vi "RT_Proof of Concept(Str).vi"() -> ()   [LabVIEW 2010]
uses:
  <vilib>/Utility/error.llb/DialogType.ctl
  <vilib>/Pansino Software/LabVIEW Architecture/PSARC_Queue Management.llb/PSARC_Queue Insert Element.vi
panel:
  out "Error Report":string
  in  "Exit":bool
  in  "OK":bool
  out "Current State":string
  in  "Temp Variable":cluster{"Error":errorcluster, "Exit":bool}
  # "————————————————\nYou could add your temporary variables\nhere.\nThis Control should be saved as a\nvi in your project folder,The proposed vi's block diagram is shown in the picture\n\n\n\n\n\n\n\n————————————————"
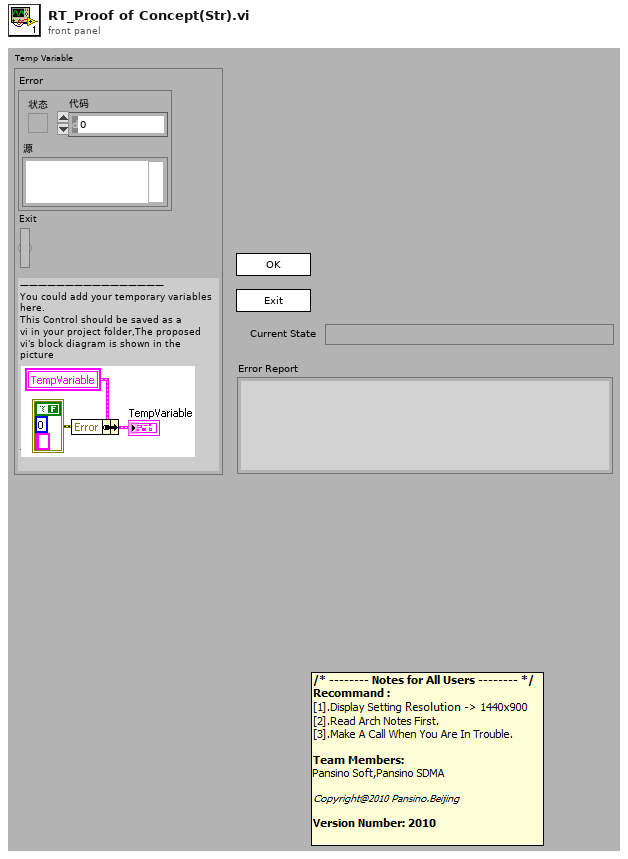
[diagram p1: front panel]
types:
  T1 = typedef "DialogType.ctl" = u16
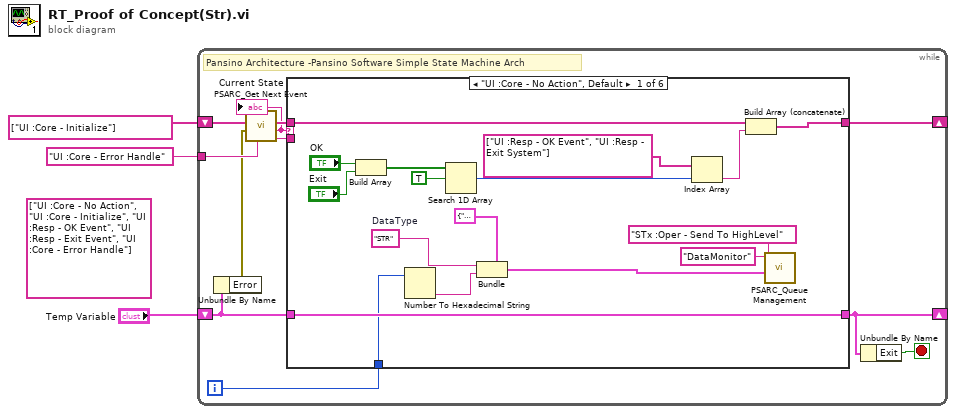
[diagram p0: block diagram]
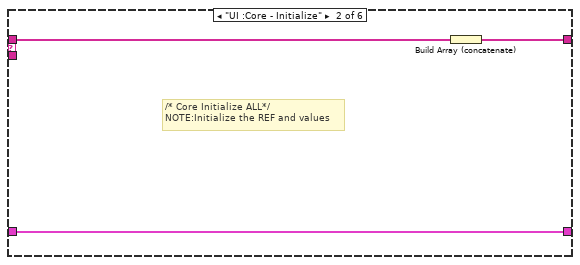
[diagram p2: hidden frame]
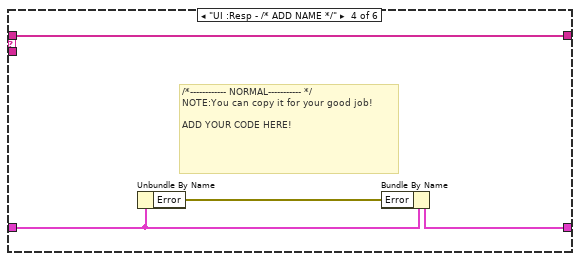
[diagram p4: hidden frame]
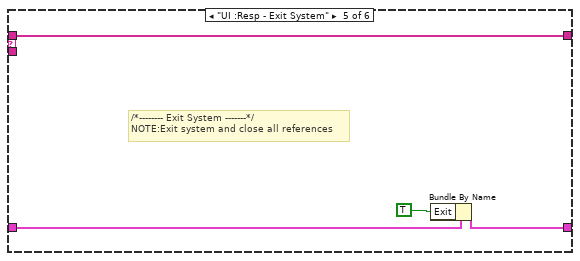
[diagram p5: hidden frame]
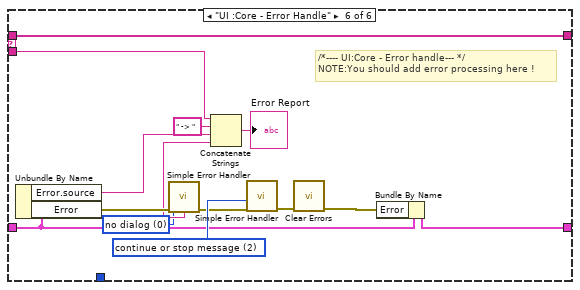
[diagram p6: hidden frame]
diagram:
  (unwired) string[] ["UI :Core - No Action", "UI :Core - Initialize", "UI :Resp - OK Event", "UI :Resp - Exit Event", "UI :Core - Error Handle"]
  n1 = while {
    tunnel: "UI :Core - Error Handle" ("Error Handle") -> [w13]
    shift-right: [w11] -> _
    shift-left: string[] ["UI :Core - Initialize"] -> [w14]
    shift-right: [w8] -> _
    shift-left: "Temp Variable" -> [w10]
    i -> [w4]
    stop <- w7 stop-if-true
    # "Pansino Architecture -Pansino Software Simple State Machine Arch"
    n2 = Unbundle By Name(w10) -> ("Error"=w9:errorcluster)
    n3 = call <vilib>:"PSARC_Get Next Event.vi"("Error Handle"=w13, "error in (no error)"=w9, "event queue in"=w14) -> ("prev event"=w5:string, "next event"=w6:string, "event queue out"=w12:string[])  [unwired: 3 in]
    "Current State" <- w6
    n4 = case shown="\"UI :Core - No Action\", Default" w6 {
      tunnel: w12 -> [w24 w34 w36 w40 w44 w58]
      tunnel: [w23 w32 w36 w40 w44 w58] -> w11
      tunnel: w10 -> [w31 w33 w35 w39 w43 w55]
      tunnel: [w31 w33 w35 w38 w42 w54] -> w8
      tunnel: w5 -> [_ _ _ _ _ w47]
      tunnel: w4 -> [w16 _ _ _ _ _]
      frame "UI :Core - No Action", Default {
        w18 = "STR"  # DataType
        n5 = Build Array("OK", "Exit") -> (w28:bool[])
        n6 = Number To Hexadecimal String(2:w16) -> (0:w15:string)  [unwired: 1 in]
        n7 = Search 1D Array(1D array=w28, element=TRUE ("元素")) -> (index of element=w25:i32)  [unwired: 1 in]
        n8 = Bundle(cluster=cluster{"DataType":string, "Data":variant} {"DataType"="", "Data"=variant}, "DataType"=w18, "Data"=w15) -> (w19:cluster{"DataType":string, "Data":variant})
        n9 = Index Array(array=string[] ["UI :Resp - OK Event", "UI :Resp - Exit System"], index=w25) -> (element=w22:string)
        n10 = Build Array (concatenate)(w24, w22) -> (w23:string[])
        n11 = call-poly <vilib>:"PSARC_Queue Management.vi"("Data"=w19, "Event"="STx :Oper - Send To HighLevel", "Queue Name(unamed)"="DataMonitor") -> ()  [unwired: 7 in, 2 out]
      }
      frame "UI :Core - Initialize" {
        # "/* Core Initialize ALL*/\nNOTE:Initialize the REF and values"
        n12 = Build Array (concatenate)(w34) -> (w32:string[])
      }
      frame "UI :Resp - OK Event" {
      }
      frame "UI :Resp - /* ADD NAME */" {
        # "/*------------ NORMAL----------- */\nNOTE:You can copy it for your good job!\n\nADD YOUR CODE HERE!"
        n13 = Unbundle By Name(w39) -> ("Error"=w37:errorcluster)
        n14 = Bundle By Name(cluster=w39, "Error"=w37) -> (w38:cluster{"Error":errorcluster, "Exit":bool})
      }
      frame "UI :Resp - Exit System" {
        # "/*-------- Exit System -------*/\nNOTE:Exit system and close all references"
        n15 = Bundle By Name(cluster=w43, "Exit"=TRUE) -> (w42:cluster{"Error":errorcluster, "Exit":bool})
      }
      frame "UI :Core - Error Handle" {
        w45 = T1 0 items=["no dialog", "OK message", "continue or stop message", "OK message + warnings", "continue/stop + warnings"] ("type of dialog (OK msg:1)")
        w57 = T1 2 items=["no dialog", "OK message", "continue or stop message", "OK message + warnings", "continue/stop + warnings"] ("type of dialog (OK msg:1)")
        # "/*---- UI:Core - Error handle--- */\nNOTE:You should add error processing here !"
        n16 = Unbundle By Name(w55) -> ("Error.source"=w51:string, "Error"=w52:errorcluster)
        n17 = call <vilib>:"Simple Error Handler.vi"("type of dialog (OK msg:1)"=w45, "error in (no error)"=w52) -> ("error out"=w50:errorcluster, "message"=w49:string)  [unwired: 3 in, 3 out]
        n18 = Concatenate Strings(w47, " -> " ("字符串"), w51, w49) -> (→"Error Report":string)
        n19 = call <vilib>:"Simple Error Handler.vi"("type of dialog (OK msg:1)"=w57, "error in (no error)"=w50) -> ("error out"=w56:errorcluster)  [unwired: 3 in, 4 out]
        n20 = call <vilib>:"Clear Errors.vi"("error in (no error)"=w56) -> ("error out"=w53:errorcluster)  [unwired: 6 in]
        n21 = Bundle By Name(cluster=w55, "Error"=w53) -> (w54:cluster{"Error":errorcluster, "Exit":bool})
      }
    }
    n22 = Unbundle By Name(w8) -> ("Exit"=w7:bool)
  }
